vi "test_TCP Write.vi"(8 "error in (no error)":errorcluster, 11 "TestCase in":refnum<class "Instrument Addon Ethernet Protocol Unit Tests.lvclass">) -> (0 "error out":errorcluster, 3 "TestCase out":refnum<class "Instrument Addon Ethernet Protocol Unit Tests.lvclass">)   [LabVIEW 2023, in "Instrument Addon Ethernet Protocol Unit Tests.lvclass"]
uses:
  Instrument Addon Ethernet Protocol Unit Tests.lvclass
  <vilib>/addons/_JKI Toolkits/VI Tester/TestCase.llb/TestCase.lvclass
  TCP/TCP.lvclass
  Constants.vi
  Listener/Listener.lvclass
  Listener/ListenerClassControls/Operation.ctl
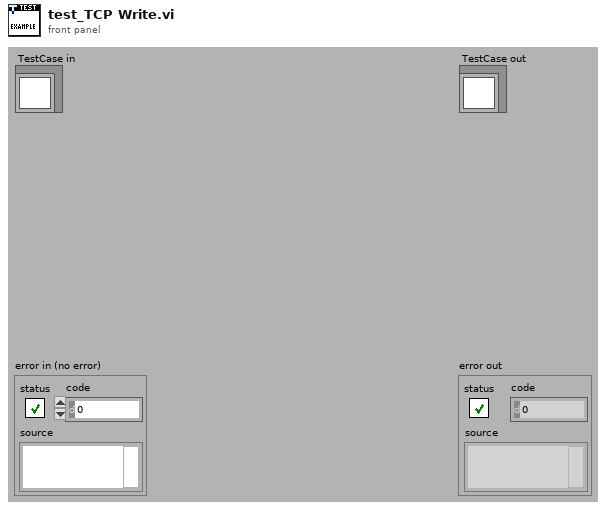
[diagram p1: front panel]
types:
  T1 = typedef "Listener.lvclass/Operation.ctl" = enum16{"Read", "Write"}
  T2 = typedef "Listener.lvclass/TCP Data Structure.ctl" = cluster{"TCP|IP connection ID":refnum<k5>, "IP Address":string, "Port":u16, "Data":string}
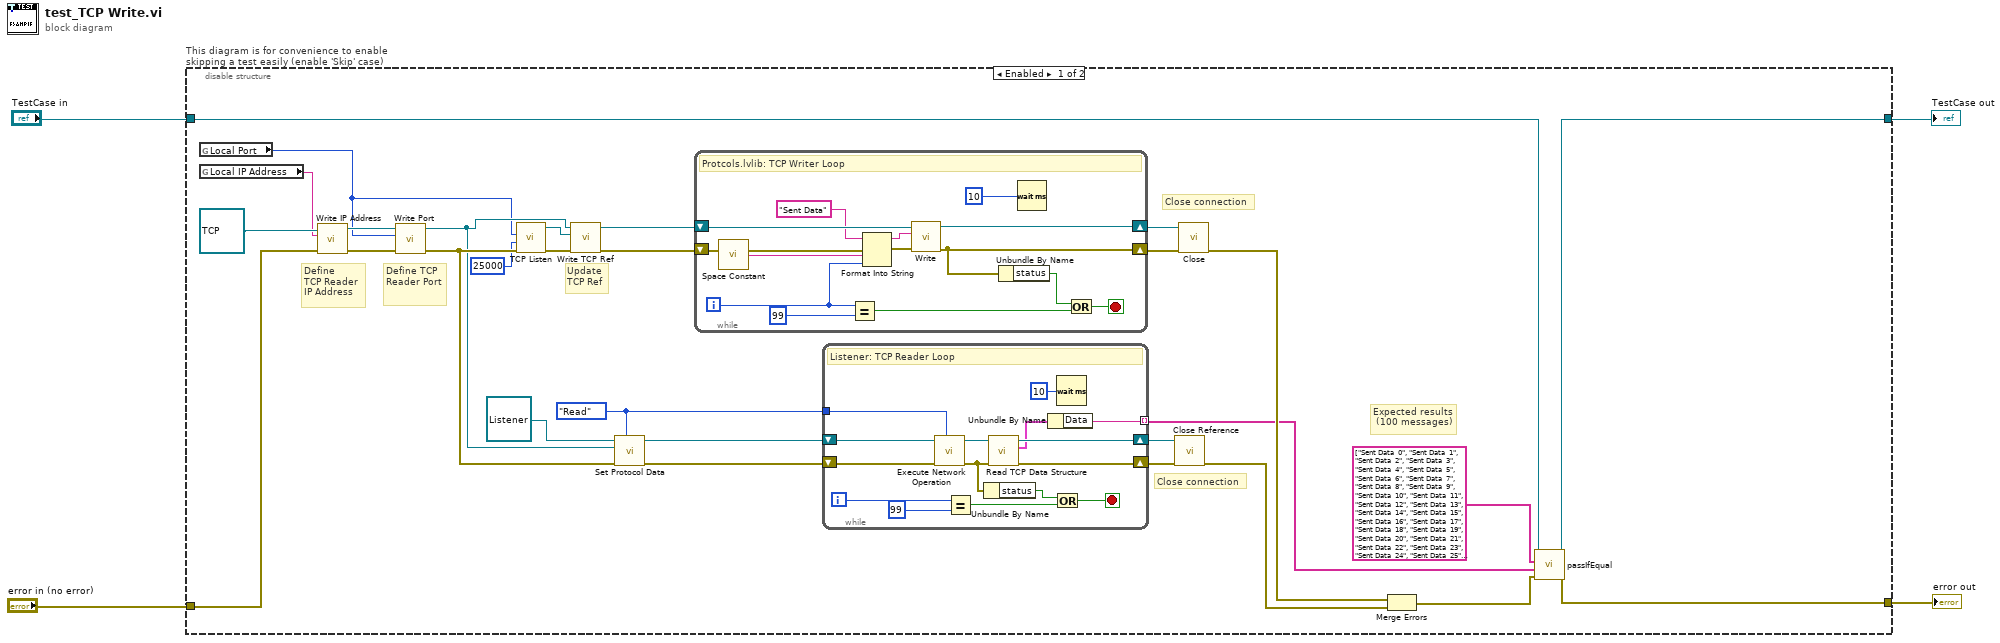
[diagram p0: block diagram]
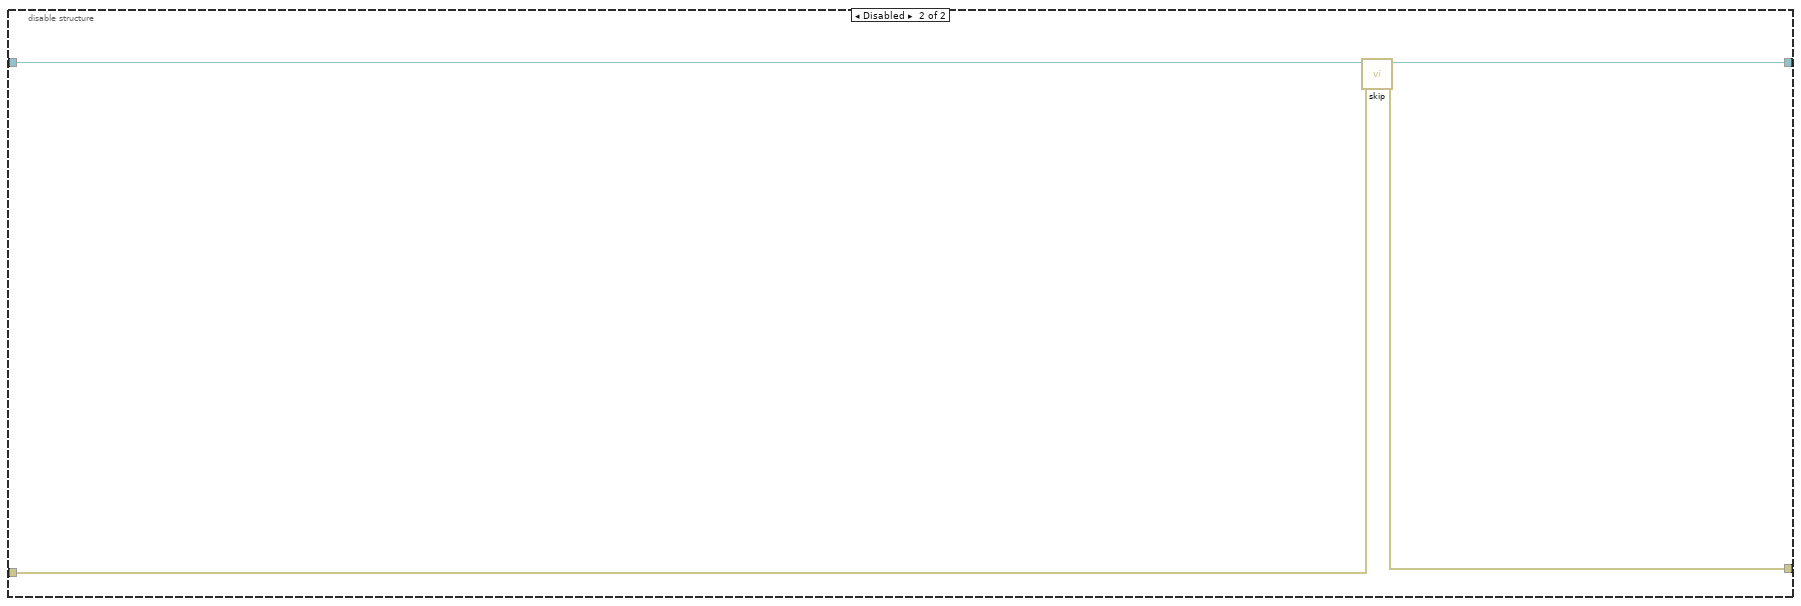
[diagram p2: hidden frame]
diagram:
  n1 = disable-structure "This diagram is for convenience to enable skipping a test easily (enable 'Skip' case)" shown="Enabled" {
    disable-tunnel: "TestCase in" -> [w33 w66]
    disable-tunnel: [w32 w64] -> w1
    disable-tunnel: [w31 w65] -> w3
    disable-tunnel: "error in (no error)" -> [w28 w63]
    frame Enabled {
      w16 = Operation."Read" ("Operation")
      # "Close connection"
      # "Close connection"
      # "Update \nTCP Ref"
      # "Expected results\n (100 messages)"
      # "Define TCP \nReader Port"
      # "Define \nTCP Reader \nIP Address"
      n2 = global read "Constants.vi" "Local Port"() -> (w5:u16)
      n3 = global read "Constants.vi" "Local IP Address"() -> (w6:string)
      n4 = call "Write IP Address.vi"("error in (no error)"=w28, "IP Address"=w6, "Ethernet in"=refnum<class "TCP.lvclass"> refnum ("Protocols.lvlib:TCP.lvclass")) -> ("error out"=w29:errorcluster, "Ethernet out"=w30:refnum<class "TCP.lvclass">)  [unwired: 7 in]
      n5 = call "Write Port.vi"("error in (no error)"=w29, "Port"=w5, "Ethernet in"=w30) -> ("error out"=w23:errorcluster, "Ethernet out"=w18:refnum<class "TCP.lvclass">)  [unwired: 7 in]
      n6 = call <vilib>:"TCP Listen.vi"("error in (no error)"=w23, "timeout ms (wait forever: -1)"=25000, "port"=w5) -> ("error out"=w21:errorcluster, "connection ID"=w17:refnum<k5>)  [unwired: 4 in, 3 out]
      n7 = call "Write TCP Ref.vi"("error in (no error)"=w21, "TCP Ref"=w17, "Ethernet in"=w18) -> ("error out"=w20:errorcluster, "Ethernet out"=w19:refnum<class "TCP.lvclass">)  [unwired: 7 in]
      n8 = call "Set Protocol Data.vi"("Operation"=w16, "error in (no error)"=w23, "Protocols.lvlib:Protocol Parent.lvclass"=w18, "Listener In.lvclass"=refnum<class "Listener.lvclass"> refnum ("Listener.lvclass")) -> ("error out"=w24:errorcluster, "Listener Out.lvclass"=w25:refnum<class "Listener.lvclass">)  [unwired: 6 in]
      n9 = while {
        shift-right: [w58] -> w12
        shift-left: w20 -> [w54]
        shift-right: [w57] -> w11
        shift-left: w19 -> [w59]
        i -> [w49]
        stop <- w61 stop-if-true
        # "Protcols.lvlib: TCP Writer Loop"
        n10 = call <vilib>:"Space Constant.vi"() -> ("String"=w53:string)
        n11 = Equal?(x=w49, y=99 ("x")) -> (x = y?=w62:bool)
        n12 = Format Into String(initial string="Sent Data" ("String"), error in=w54, w53, w49) -> (resulting string=w51:string, error out=w52:errorcluster)  [unwired: 1 in]
        n13 = call-dynamic "Write.vi"("error in (no error)"=w52, "String"=w51, "Ethernet in"=w59) -> ("error out"=w58:errorcluster, "Ethernet out"=w57:refnum<class "TCP.lvclass">)  [unwired: 7 in]
        n14 = Unbundle By Name(w58) -> ("status"=w56:bool)
        n15 = Wait (ms)(milliseconds to wait=u32 10) -> ()  [unwired: 1 out]
        n16 = Or(x=w56, y=w62) -> (x .or. y?=w61:bool)
      }
      n17 = while {
        shift-right: [w35] -> w14
        shift-left: w24 -> [w48]
        shift-right: [w36] -> w15
        shift-left: w25 -> [w47]
        tunnel: w16 -> [w42]
        tunnel: [w41] -> w9 mode=indexing
        i -> [w40]
        stop <- w45 stop-if-true
        # "Listener: TCP Reader Loop"
        n18 = call "Execute Network Operation.vi"("Operation"=w42, "error in (no error)"=w48, "Listener In.lvclass"=w47) -> ("error out"=w38:errorcluster, "Listener Out.lvclass"=w37:refnum<class "Listener.lvclass">)  [unwired: 7 in]
        n19 = Equal?(x=w40, y=99 ("x")) -> (x = y?=w44:bool)
        n20 = Unbundle By Name(w38) -> ("status"=w46:bool)
        n21 = call-dynamic "Read TCP Data Structure.vi"("error in (no error)"=w38, "Listener in"=w37) -> ("error out"=w35:errorcluster, "TCP|IP Data Structure"=w34:T2, "Listener out"=w36:refnum<class "Listener.lvclass">)  [unwired: 7 in]
        n22 = Unbundle By Name(w34) -> ("Data"=w41:string)
        n23 = Or(x=w46, y=w44) -> (x .or. y?=w45:bool)
        n24 = Wait (ms)(milliseconds to wait=u32 10) -> ()  [unwired: 1 out]
      }
      n25 = call "Close Reference.vi"("error in (no error)"=w14, "Listener In.lvclass"=w15) -> ("error out"=w13:errorcluster)  [unwired: 8 in, 1 out]
      n26 = call-dynamic "Close.vi"("error in (no error)"=w12, "Ethernet in"=w11) -> ("error out"=w10:errorcluster)  [unwired: 8 in, 1 out]
      n27 = Merge Errors(w10, w13) -> (w27:errorcluster)
      n28 = call-dynamic "passIfEqual.vi"("error in (no error)"=w27, "y"=w9, "x"=string[] ["Sent Data  0", "Sent Data  1", "Sent Data  2", "Sent Data  3", "Sent Data  4", "Sent Data  5", "Sent Data  6", "Sent Data  7", "Sent Data  8", "Sent Data  9", "Sent Data  10", "Sent Data  11", "Sent Data  12", "Sent Data  13", "Sent Data  14", "Sent Data  15", "Sent Data  16", "Sent Data  17", "Sent Data  18", "Sent Data  19", "Sent Data  20", "Sent Data  21", "Sent Data  22", "Sent Data  23", "Sent Data  24", "Sent Data  25", "Sent Data  26", "Sent Data  27", "Sent Data  28", "Sent Data  29", "Sent Data  30", "Sent Data  31", "Sent Data  32", "Sent Data  33", "Sent Data  34", "Sent Data  35", "Sent Data  36", "Sent Data  37", "Sent Data  38", "Sent Data  39", "Sent Data  40", "Sent Data  41", "Sent Data  42", "Sent Data  43", "Sent Data  44", "Sent Data  45", "Sent Data  46", "Sent Data  47", "Sent Data  48", "Sent Data  49", "Sent Data  50", "Sent Data  51", "Sent Data  52", "Sent Data  53", "Sent Data  54", "Sent Data  55", "Sent Data  56", "Sent Data  57", "Sent Data  58", "Sent Data  59", "Sent Data  60", "Sent Data  61", "Sent Data  62", "Sent Data  63", "Sent Data  64", "Sent Data  65", "Sent Data  66", "Sent Data  67", "Sent Data  68", "Sent Data  69", "Sent Data  70", "Sent Data  71", "Sent Data  72", "Sent Data  73", "Sent Data  74", "Sent Data  75", "Sent Data  76", "Sent Data  77", "Sent Data  78", "Sent Data  79", "Sent Data  80", "Sent Data  81", "Sent Data  82", "Sent Data  83", "Sent Data  84", "Sent Data  85", "Sent Data  86", "Sent Data  87", "Sent Data  88", "Sent Data  89", "Sent Data  90", "Sent Data  91", "Sent Data  92", "Sent Data  93", "Sent Data  94", "Sent Data  95", "Sent Data  96", "Sent Data  97", "Sent Data  98", "Sent Data  99"] ("Array"), "TestCase in"=w33) -> ("error out"=w31:errorcluster, "TestCase out"=w32:refnum<class "Instrument Addon Ethernet Protocol Unit Tests.lvclass">)  [unwired: 6 in]
    }
    frame Disabled {
      # "skip test result while test is under development"
      n29 = call <vilib>:"skip.vi"("error in (no error)"=w63, "TestCase in"=w66) -> ("error out"=w65:errorcluster, "TestCase out"=w64:refnum<class "Instrument Addon Ethernet Protocol Unit Tests.lvclass">)  [unwired: 8 in]
    }
  }
  "error out" <- w3
  "TestCase out" <- w1
